vi "Main.vi"() -> ()   [LabVIEW 2020]
uses:
  TypeDefs/Control_MaquinaEstados.ctl
  <vilib>/Utility/error.llb/DialogType.ctl
  <vilib>/numeric/Random Number (Range) DBL.vi
  <vilib>/JKI/JKI Simple Localization/API/JKI Simple LocalizationJKI_Simple_Localization.lvlib
  <vilib>/Utility/SystemLogging/NI_SystemLogging.lvlib
  <vilib>/JKI/JKI Simple Localization/Private/RegisterVIJKI_Simple_Localization.vi
panel:
  in  "View Button":bool
  out "error out":errorcluster
  in  "Language":enum32{"Button 1", "Button 2"}(radio)
  in  "DIctionary":path
  out "Current Language":string
  out "notification 4":bool
  out "notification 3":bool
  out "notification 2":bool
  out "notification":bool
  out "Tab Control":enum32{"Page 1", "Page 2", "Page 3"}(tab)
  in  "Start Button":bool
  in  "Path Control":path=path "C:/Users/Israel MACIAS/Desktop/Proyecto.bmp"
  in  "Save Tool":bool
  out "Waveform Chart - Dark":dbl(graph)
  in  "Tabs Buttons":enum32{"Button 1", "Button 2", "Button 3"}(radio)
  in  "Abort Button":bool
  # "Debbugging Additional Objets"
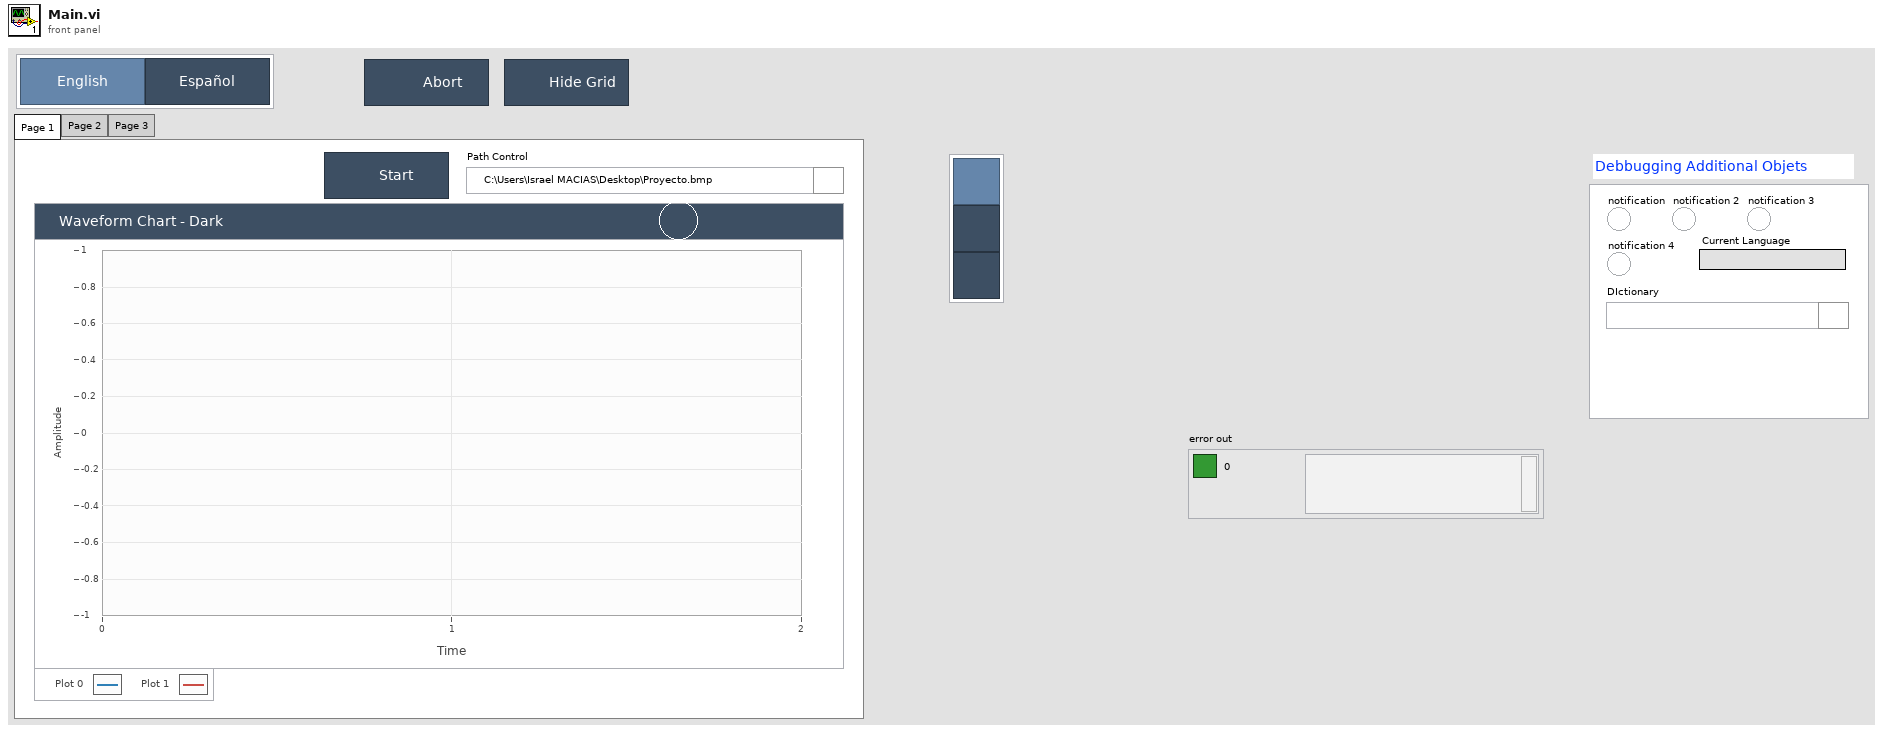
[diagram p1: front panel]
types:
  T1 = typedef "Control_MaquinaEstados.ctl" = enum16{"Starting up", "Adquisition", "Save", "Fault"}
  T2 = typedef "DialogType.ctl" = u16
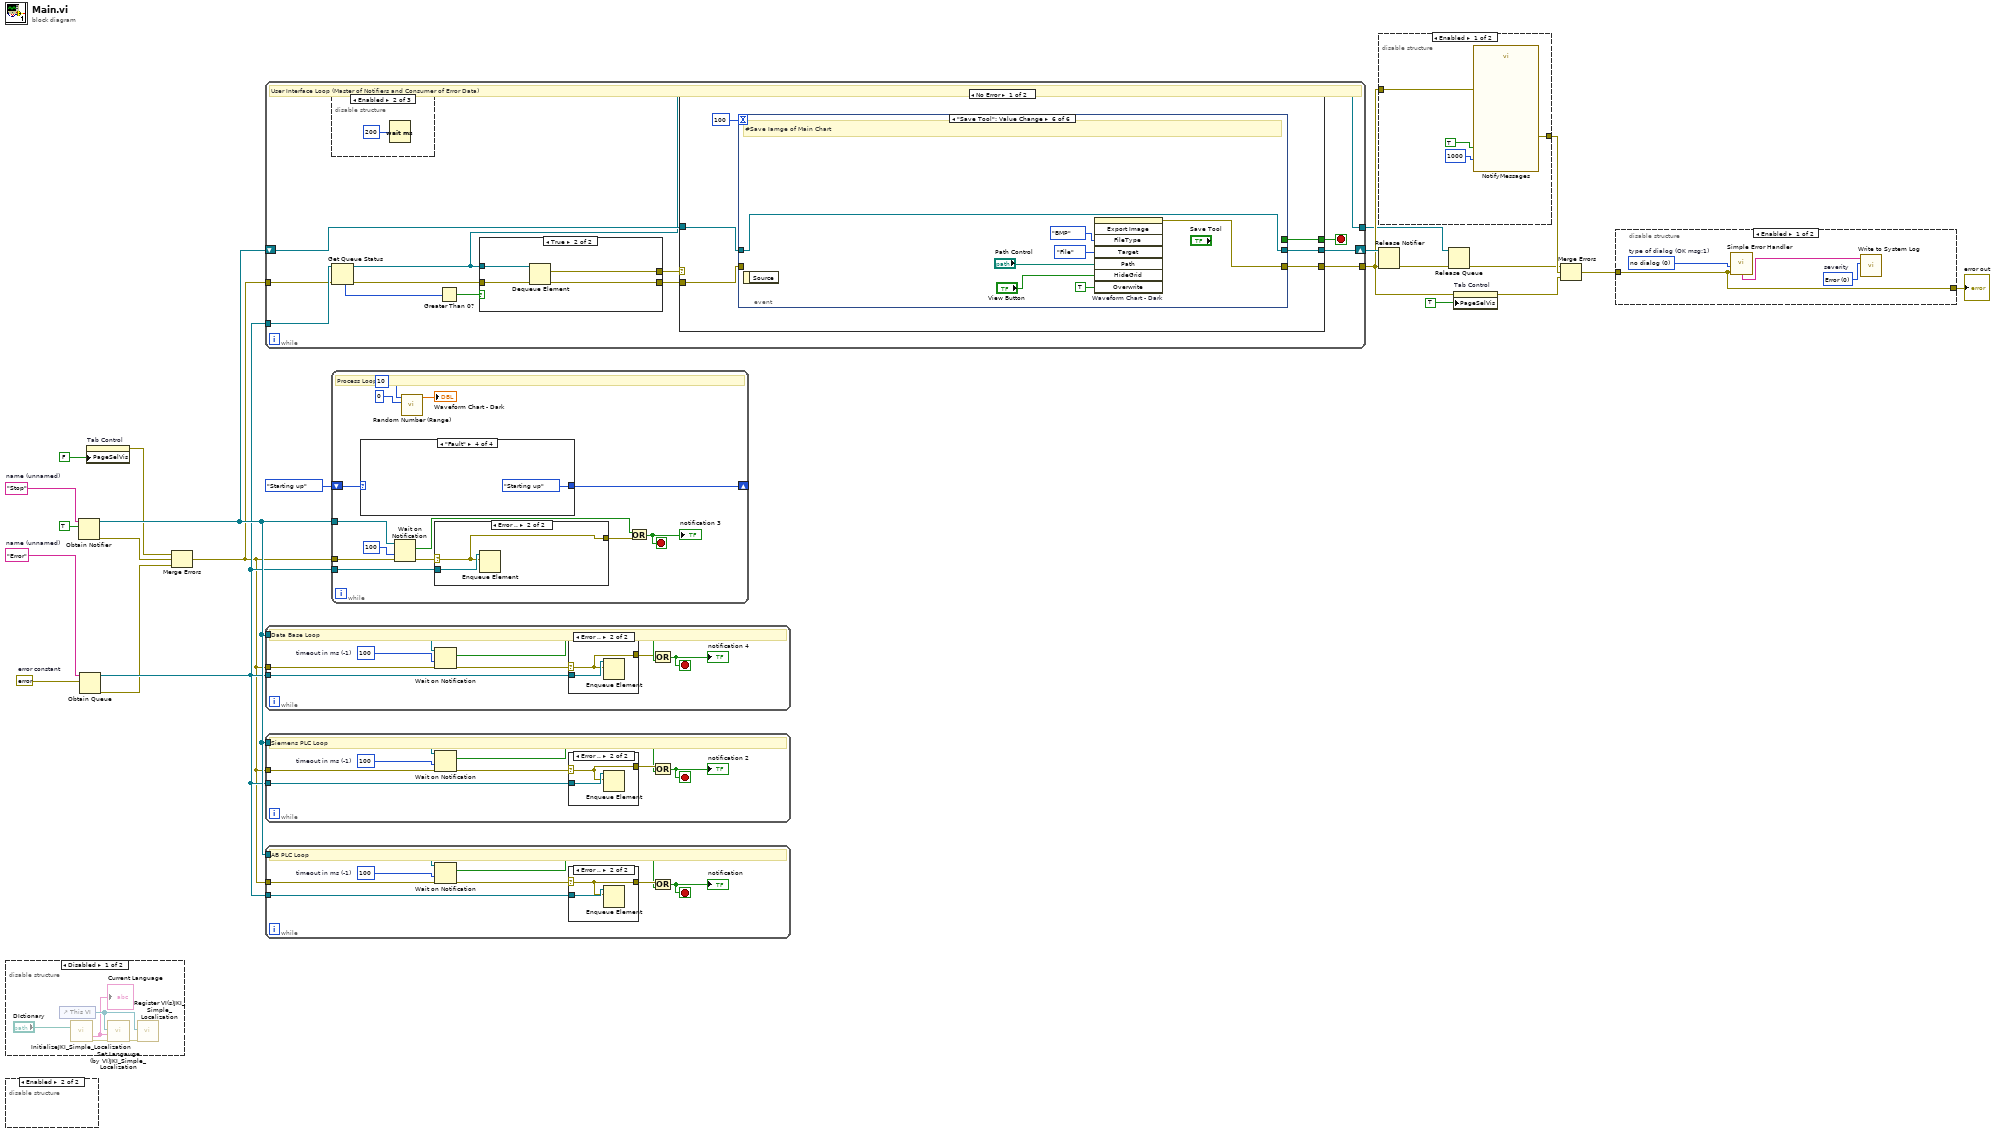
[diagram p0: block diagram]
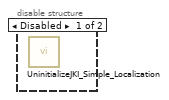
[diagram p4: hidden frame]
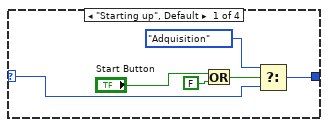
[diagram p7: hidden frame]
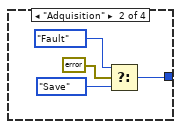
[diagram p8: hidden frame]
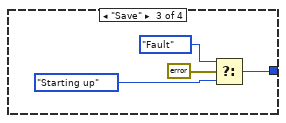
[diagram p9: hidden frame]
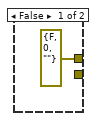
[diagram p13: hidden frame]
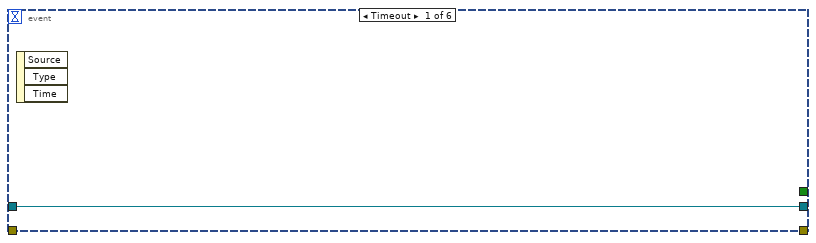
[diagram p14: hidden frame]
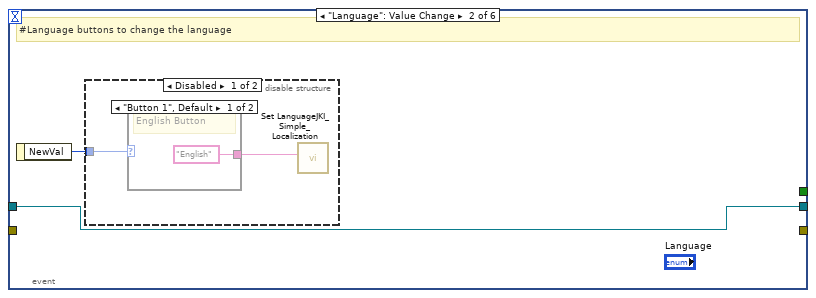
[diagram p15: hidden frame]
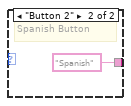
[diagram p16: hidden frame]
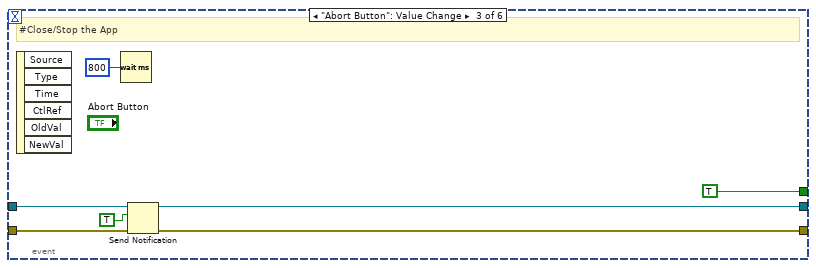
[diagram p18: hidden frame]
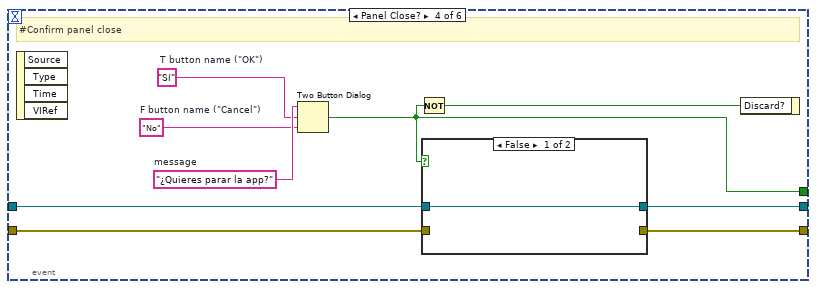
[diagram p19: hidden frame]
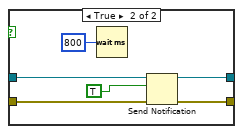
[diagram p20: hidden frame]
diagram:
  w17 = errorcluster {"status"=FALSE, "code"=0, "source"=""}  # error constant
  w18 = "Error"  # name (unnamed)
  w22 = "Stop"  # name (unnamed)
  n1 = disable-structure "Diagram Disable Structure" shown="Disabled" {
    frame Disabled {
      n2 = control-ref of="This VI"() -> (w24:refnum<vi>)
      n3 = call <vilib>:"InitializeJKI_Simple_Localization.vi"("Dictionary File Path"="DIctionary") -> ("Current Language"=w23:string, "error out"=w26:errorcluster)  [unwired: 11 in, 2 out]
      "Current Language" <- w23
      n4 = call <vilib>:"Set Langauge (by VI)JKI_Simple_Localization.vi"("error in"=w26, "Target Language"=w23, "VI Ref"=w24) -> ("error out"=w25:errorcluster)  [unwired: 8 in]
      n5 = call-poly <vilib>:"Register VI(s)JKI_Simple_Localization.vi"("error in"=w25, "VI Ref"=w24) -> ()  [unwired: 8 in, 2 out]
    }
    frame Enabled {
    }
  }
  n6 = disable-structure "Diagram Disable Structure" shown="Enabled" {
    frame Disabled {
      n7 = call <vilib>:"UninitializeJKI_Simple_Localization.vi"() -> ()  [unwired: 11 in, 1 out]
    }
    frame Enabled {
    }
  }
  n8 = Obtain Notifier(name (unnamed)=w22, notification data type=TRUE) -> (notifier out=w19:refnum<notifier>, error out=w14:errorcluster)  [unwired: 2 in, 1 out]
  n9 = Obtain Queue(name (unnamed)=w18, element data type=w17) -> (queue out=w16:refnum<queue>, error out=w15:errorcluster)  [unwired: 3 in, 1 out]
  n10 = property on="Tab Control" class="TabCtl (strict)"("PageSelVis"=FALSE ("Page Selector Visible")) -> (error out=w9:errorcluster)  [unwired: 2 in, 1 out]
  n11 = Merge Errors "Merge Errors"(w9, w14, w15) -> (w13:errorcluster)
  n12 = while {
    shift-right: [w38] -> w20
    shift-left: w19 -> [w37]
    tunnel: w16 -> [w34]
    tunnel: w13 -> [w31]
    tunnel: [w35] -> w5
    tunnel: [w28] -> w2
    stop <- w39 stop-if-true
    # "User Interface Loop (Master of Notifiers and Consumer of Error Data)"
    n13 = disable-structure shown="Enabled" {
      frame Disabled {
      }
      frame Enabled {
        n14 = Wait (ms)(milliseconds to wait=u32 200 ("millisecond multiple")) -> ()  [unwired: 1 out]
      }
      frame Disabled {
      }
    }
    n15 = Get Queue Status(queue=w34, error in (no error)=w31) -> (queue out=w28:refnum<queue>, error out=w30:errorcluster, # elements in queue=w32:i32)  [unwired: 1 in, 5 out]
    n16 = Greater Than 0?(x=w32) -> (x > 0?=w33:bool)
    n17 = case shown="True" w33 {
      tunnel: [errorcluster {"status"=FALSE, "code"=0, "source"=""} ("error constant") w44] -> w36
      tunnel: w28 -> [_ w43]
      tunnel: w30 -> [_ w42]
      tunnel: [_ w41] -> w29
      frame False {
      }
      frame True {
        n18 = Dequeue Element(queue=w43, error in (no error)=w42) -> (element=w44:errorcluster, error out=w41:errorcluster)  [unwired: 1 in, 2 out]
      }
    }
    n19 = case shown="No Error" w36 {
      selector: w36 -> [_ w92]
      tunnel: [w50 TRUE ("T button?")] -> w39
      tunnel: [w49 w95] -> w38
      tunnel: w37 -> [w48 w98]
      tunnel: w29 -> [w46 _]
      tunnel: [w45 w91] -> w35
      frame No Error {
        n20 = event shown="[5] \"Save Tool\": Value Change" {
          selector: _ -> [_ _ _ _ _ _]
          dyn-events: _ -> [_ _ _ _ _ _]
          timeout: 100 -> [_ _ _ _ _ _]
          tunnel: [_ _ TRUE ("Abort Button") w69 _ _] -> w50
          tunnel: w48 -> [w51 w52 w63 w68 w81 w85]
          tunnel: [w51 w52 w60 w67 w81 w85] -> w49
          tunnel: w46 -> [_ _ w59 w65 _ _]
          tunnel: [_ _ w58 w66 _ w86] -> w45
          event Timeout {
            n21 = event-data() -> ()  [unwired: 1 in, 3 out]
          }
          event "Language": Value Change {
            # "#Language buttons to change the language"
            n22 = event-data() -> ("NewVal"=w53:enum32{"Button 1", "Button 2"})  [unwired: 1 in]
            n23 = disable-structure shown="Disabled" {
              disable-tunnel: w53 -> [w54 _]
              frame Disabled {
                n24 = case shown="\"Button 1\", Default" w54 {
                  tunnel: ["English" ("Target Language") "Spanish" ("Target Language")] -> w55
                  frame "Button 1", Default {
                    # "English Button"
                  }
                  frame "Button 2" {
                    # "Spanish Button"
                  }
                }
                n25 = call <vilib>:"Set LanguageJKI_Simple_Localization.vi"("Target Language (current lang)"=w55) -> ()  [unwired: 9 in, 2 out]
              }
              frame Enabled {
              }
            }
          }
          event "Abort Button": Value Change {
            # "#Close/Stop the App"
            n26 = event-data() -> ()  [unwired: 1 in, 6 out]
            n27 = Wait (ms)(milliseconds to wait=u32 800) -> ()  [unwired: 1 out]
            n28 = Send Notification(notification=TRUE, notifier=w63, error in (no error)=w59) -> (notifier out=w60:refnum<notifier>, error out=w58:errorcluster)
          }
          event Panel Close? {
            w71 = "No"  # F button name ("Cancel")
            w72 = "Sí"  # T button name ("OK")
            w73 = "¿Quieres parar la app?"  # message
            # "#Confirm panel close"
            n29 = event-data() -> ()  [unwired: 1 in, 4 out]
            n30 = Two Button Dialog(message=w73, 1:w71, 2:w72) -> (T button?=w69:bool)
            n31 = Not(x=w69) -> (.not. x?=w70:bool)
            n32 = case shown="False" w69 {
              tunnel: w68 -> [w74 w80]
              tunnel: [w74 w77] -> w67
              tunnel: [_ w76] -> w66
              tunnel: w65 -> [_ w75]
              frame False {
              }
              frame True {
                n33 = Wait (ms)(milliseconds to wait=u32 800) -> ()  [unwired: 1 out]
                n34 = Send Notification(notification=TRUE, notifier=w80, error in (no error)=w75) -> (notifier out=w77:refnum<notifier>, error out=w76:errorcluster)
              }
            }
            n35 = event-data("Discard?"=w70) -> ()  [unwired: 1 in, 1 out]
          }
          event "Tabs Buttons": Value Change {
            # "#Tabs Buttons"
            n36 = event-data() -> ("NewVal"=w83:enum32{"Button 1", "Button 2", "Button 3"})  [unwired: 1 in, 2 out]
            n37 = To Word Integer(number=w83) -> (16bit integer=→"Tab Control":i16)
          }
          event "Save Tool": Value Change {
            # "#Save Iamge of Main Chart"
            n38 = event-data() -> ()  [unwired: 1 in, 1 out]
            n39 = invoke on="Waveform Chart - Dark" class="WFChart (strict)" method="Export Image"("FileType"=enum32{"BMP", "EPS", "EMF", "PICT"}."BMP" ("File Type"), "Target"=enum32{"File", "Clipboard"}."File", "Path"="Path Control", "HideGrid"="View Button", "Overwrite"=TRUE ("Always Overwrite")) -> (error out=w86:errorcluster)  [unwired: 3 in, 7 out]
          }
        }
      }
      frame Error {
        n40 = Wait (ms)(milliseconds to wait=u32 800) -> ()  [unwired: 1 out]
        n41 = Send Notification(notification=TRUE, notifier=w98) -> (notifier out=w95:refnum<notifier>, error out=w93:errorcluster)  [unwired: 1 in]
        n42 = Merge Errors "Merge Errors"(w93, w92) -> (w91:errorcluster)
      }
    }
  }
  n43 = while {
    tunnel: w19 -> [w107]
    tunnel: w16 -> [w105]
    tunnel: w13 -> [w104]
    stop <- w100 stop-if-true
    w106 = 100  # timeout in ms (-1)
    # "Data Base Loop"
    n44 = Wait on Notification(notifier=w107, timeout in ms (-1)=w106, error in (no error)=w104) -> (notification=w102:bool, error out=w103:errorcluster)  [unwired: 1 in, 2 out]
    n45 = case shown="Error .." w103 {
      selector: w103 -> [_ w108]
      tunnel: w105 -> [_ w109]
      tunnel: [_ w108] -> w101
      frame No Error {
      }
      frame Error {
        n46 = Enqueue Element(queue=w109, element=w108) -> ()  [unwired: 2 in, 3 out]
      }
    }
    n47 = Or(x=w101, y=w102) -> (x .or. y?=w100:bool)
    "notification 4" <- w100
  }
  n48 = while {
    tunnel: w19 -> [w117]
    tunnel: w16 -> [w115]
    tunnel: w13 -> [w114]
    stop <- w110 stop-if-true
    w116 = 100  # timeout in ms (-1)
    # "Siemens PLC Loop"
    n49 = Wait on Notification(notifier=w117, timeout in ms (-1)=w116, error in (no error)=w114) -> (notification=w111:bool, error out=w113:errorcluster)  [unwired: 1 in, 2 out]
    n50 = case shown="Error .." w113 {
      selector: w113 -> [_ w118]
      tunnel: w115 -> [_ w119]
      tunnel: [_ w118] -> w112
      frame No Error {
      }
      frame Error {
        n51 = Enqueue Element(queue=w119, element=w118) -> ()  [unwired: 2 in, 3 out]
      }
    }
    n52 = Or(x=w112, y=w111) -> (x .or. y?=w110:bool)
    "notification 2" <- w110
  }
  n53 = while {
    tunnel: w19 -> [w127]
    tunnel: w16 -> [w125]
    tunnel: w13 -> [w123]
    stop <- w120 stop-if-true
    w126 = 100  # timeout in ms (-1)
    # "AB PLC Loop"
    n54 = Wait on Notification(notifier=w127, timeout in ms (-1)=w126, error in (no error)=w123) -> (notification=w121:bool, error out=w124:errorcluster)  [unwired: 1 in, 2 out]
    n55 = case shown="Error .." w124 {
      selector: w124 -> [_ w128]
      tunnel: w125 -> [_ w129]
      tunnel: [_ w128] -> w122
      frame No Error {
      }
      frame Error {
        n56 = Enqueue Element(queue=w129, element=w128) -> ()  [unwired: 2 in, 3 out]
      }
    }
    n57 = Or(x=w122, y=w121) -> (x .or. y?=w120:bool)
    "notification" <- w120
  }
  n58 = while {
    tunnel: w19 -> [w142]
    tunnel: w16 -> [w140]
    tunnel: w13 -> [w139]
    shift-right: [w130] -> _
    shift-left: Control_MaquinaEstados."Starting up" ("Enum - Menu") -> [w131]
    stop <- w136 stop-if-true
    # "Process Loop"
    n59 = case shown="\"Fault\"" w131 {
      selector: w131 -> [w144 _ _ _]
      tunnel: [w143 w149 w156 Control_MaquinaEstados."Starting up" ("Enum - Menu")] -> w130
      frame "Starting up", Default {
        n60 = Or(x="Start Button", y=FALSE) -> (x .or. y?=w146:bool)
        n61 = Select(t=Control_MaquinaEstados."Adquisition" ("Enum - Menu"), s=w146, f=w144) -> (s? t:f=w143:T1)
      }
      frame "Adquisition" {
        n62 = Select(t=Control_MaquinaEstados."Fault" ("Enum - Menu"), s=errorcluster {"status"=FALSE, "code"=0, "source"=""} ("error constant"), f=Control_MaquinaEstados."Save" ("Enum - Menu")) -> (s? t:f=w149:T1)
      }
      frame "Save" {
        n63 = Select(t=Control_MaquinaEstados."Fault" ("Enum - Menu"), s=errorcluster {"status"=FALSE, "code"=0, "source"=""} ("error constant"), f=Control_MaquinaEstados."Starting up" ("Enum - Menu")) -> (s? t:f=w156:T1)
      }
      frame "Fault" {
      }
    }
    n64 = Wait on Notification(notifier=w142, timeout in ms (-1)=100, error in (no error)=w139) -> (notification=w137:bool, error out=w135:errorcluster)  [unwired: 1 in, 2 out]
    n65 = call-poly <vilib>:"Random Number (Range).vi"("lower bound (0)"=u64 0, "upper bound (100)"=u64 10) -> ("number"=→"Waveform Chart - Dark":dbl)  [unwired: 9 in]
    n66 = case shown="Error .." w135 {
      selector: w135 -> [_ w158]
      tunnel: w140 -> [_ w159]
      tunnel: [_ w158] -> w138
      frame No Error {
      }
      frame Error {
        n67 = Enqueue Element(queue=w159, element=w158) -> ()  [unwired: 2 in, 3 out]
      }
    }
    n68 = Or(x=w137, y=w138) -> (x .or. y?=w136:bool)
    "notification 3" <- w136
  }
  n69 = disable-structure "Diagram Disable Structure" shown="Enabled" {
    disable-tunnel: w5 -> [w163 _]
    disable-tunnel: [w160 _] -> w12
    frame Enabled {
      n70 = call "NotifyMessages.vi"("Add Alarm Button"=TRUE, "milliseconds to wait"=u32 1000, "error in (no error)"=w163) -> ("error out"=w160:errorcluster)  [unwired: 8 in]
    }
    frame Disabled {
    }
  }
  n71 = Release Notifier(notifier=w20, error in (no error)=w5) -> (error out=w4:errorcluster)  [unwired: 1 in, 2 out]
  n72 = Release Queue(queue=w2, error in (no error)=w4) -> (error out=w3:errorcluster)  [unwired: 1 in, 2 out]
  n73 = property on="Tab Control" class="TabCtl (strict)"(error in=w5, "PageSelVis"=TRUE ("Page Selector Visible")) -> (error out=w6:errorcluster)  [unwired: 1 in, 1 out]
  n74 = Merge Errors "Merge Errors"(w3, w12, w6) -> (w11:errorcluster)
  n75 = disable-structure "Diagram Disable Structure" shown="Enabled" {
    disable-tunnel: w11 -> [w164 _]
    disable-tunnel: [w164 _] -> w10
    frame Enabled {
      w166 = 0 items=["Error", "Warning", "Informational"]  # severity
      w167 = T2 0 items=["no dialog", "OK message", "continue or stop message", "OK message + warnings", "continue/stop + warnings"]  # type of dialog (OK msg:1)
      n76 = call <vilib>:"Simple Error Handler.vi"("type of dialog (OK msg:1)"=w167, "error in (no error)"=w164) -> ("message"=w165:string)  [unwired: 3 in, 4 out]
      n77 = call <vilib>:"Write to System Log.vi"("severity"=w166, "message"=w165) -> ()  [unwired: 9 in, 1 out]
    }
    frame Disabled {
    }
  }
  "error out" <- w10
